vi "Get Waveform Type.vi"(8 "error in (no error)":errorcluster, 11 "VISA resource name":refnum<visa-resource-name>) -> (0 "error out":errorcluster {"code" format="%.0x"}, 1 "2nd Waveform":i32, 2 "1st Waveform":i32, 3 "VISA resource name out":refnum<visa-resource-name>)   [LabVIEW 2014, in "Fluke 5XXX Series Multicalibrators.lvlib"]
doc: "This VI returns the waveform types for ac outputs. Waveform choices are SINE (sinewave), TRI (trianglewave), SQUARE (squarewave), TRUNCS (truncated sinewave), or NONE (waveform does not apply).\n\nNote:\n\nThis VI is available only for instrument models 5500A and 5520A."
uses:
  Fluke 5XXX Series Multicalibrators.lvlib
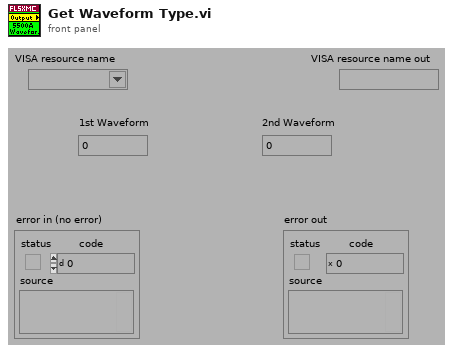
[diagram p1: front panel]
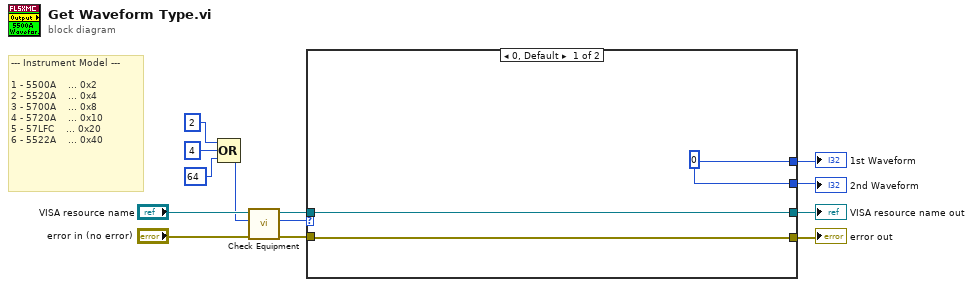
[diagram p0: block diagram]
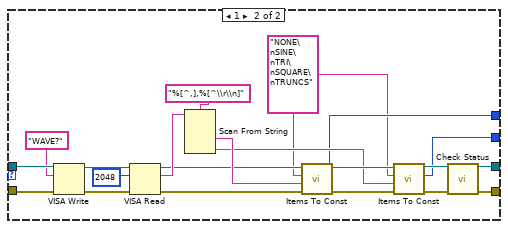
[diagram p2: hidden frame]
diagram:
  # "--- Instrument Model ---\n\n1 - 5500A    ... 0x2\n2 - 5520A    ... 0x4\n3 - 5700A    ... 0x8\n4 - 5720A    ... 0x10\n5 - 57LFC    ... 0x20\n6 - 5522A    ... 0x40"
  n1 = Compound Arithmetic op=OR(2 ("Numeric"), 4 ("Numeric"), 64 ("Numeric")) -> (w1:i32)
  n2 = call "Check Equipment.vi"("error in (no error)"="error in (no error)", "Bit Mask"=w1, "VISA resource name"="VISA resource name") -> ("error out"=w13:errorcluster, "Present?"=w12:u32, "VISA resource name out"=w11:refnum<visa-resource-name>)  [unwired: 6 in]
  n3 = case shown="0, Default" w12 {
    tunnel: [w15 w20] -> w7
    tunnel: w13 -> [w16 w37]
    tunnel: w11 -> [w15 w36]
    tunnel: [w16 w25] -> w10
    tunnel: [w14 w19] -> w6
    tunnel: [w14 w18] -> w5
    frame 0, Default {
      w14 = u16 0 ("f")
    }
    frame 1 {
      w17 = "NONE\nSINE\nTRI\nSQUARE\nTRUNCS"
      n4 = VISA Write(VISA resource name=w36, write buffer="WAVE?", error in (no error)=w37) -> (VISA resource name out=w33:refnum<visa-resource-name>, error out=w32:errorcluster)  [unwired: 1 out]
      n5 = VISA Read(VISA resource name=w33, byte count=u32 2048 ("byte count (0)"), error in (no error)=w32) -> (VISA resource name out=w22:refnum<visa-resource-name>, read buffer=w30:string, error out=w23:errorcluster)  [unwired: 1 out]
      n6 = Scan From String(format string="%[^,],%[^\\r\\n]", input string=w30) -> (output 1=w27:string, output 2=w26:string)  [unwired: 4 in, 3 out]
      n7 = call "Items To Const.vi"("error in (no error)"=w23, "String Item"=w27, "Multi-Line String"=w17, "VISA resource name"=w22) -> ("error out"=w29:errorcluster, "Index"=w19:i32, "VISA resource name out"=w28:refnum<visa-resource-name>)  [unwired: 5 in]
      n8 = call "Items To Const.vi"("error in (no error)"=w29, "String Item"=w26, "Multi-Line String"=w17, "VISA resource name"=w28) -> ("error out"=w24:errorcluster, "Index"=w18:i32, "VISA resource name out"=w21:refnum<visa-resource-name>)  [unwired: 5 in]
      n9 = call "Check Status.vi"("VISA resource name"=w21, "error in (no error)"=w24) -> ("VISA resource name out"=w20:refnum<visa-resource-name>, "error out"=w25:errorcluster)  [unwired: 12 in]
    }
  }
  "1st Waveform" <- w6
  "2nd Waveform" <- w5
  "VISA resource name out" <- w7
  "error out" <- w10
